vi "GEvt-Generate Unregister Log.vi"(0 "CSM Global Log Event":T4, 1 "Current State":string, 2 "Arguments":string, 6 "Name (\"\" to Use UUID)":string, 7 "Remove For Module Exit? (F)":bool, 10 "CSM:LogFilter.lvclass":refnum<class "LogFilter.lvclass">) -> (14 "CSM Global Log Event Out":T4, 16 "Event Data":T1={"Name (\"\" to Use UUID)"="", "Current State"="", "Arguments"="", "Source Message"={"‘State"="", "’Arguments"="", "’Error"={"status"=FALSE, "code"=0, "source"=""}}, "Source Module"="", "Complete(T)/Start(F)"=FALSE, "LogType"=enum."State Change", "Time Stamp"=timestamp(0 s since 1904-01-01)})   [LabVIEW 2017, in "Communicable State Machine.lvlib"]
doc: "### GEvt-Generate Unregister Log.vi\n\n-- <b>Controls</b> --\n- <b>CSM Global Log Event</b>:\n- <b>Current State</b>:\n- <b>Arguments</b>:\n- <b>Name(\"\" to use uuid)</b>:\n- <b>CSM:LogFilter.lvclass</b>:\n\n-- <b>Indicators</b> --\n- <b>CSM Global Log Event out</b>:\n- <b>event data</b>:"
uses:
  Communicable State Machine.lvlib
  GEvt-Refs.ctl
  Typedef/_CSM_GlobalLog_MSG.ctl
  Typedef/_CSM_Response Source Message.ctl
  Typedef/_CSM_GlobalLog_MSG_TYPE.ctl
  LogFilter/LogFilter.lvclass
  LogFilter/LogFilter - Check.vi
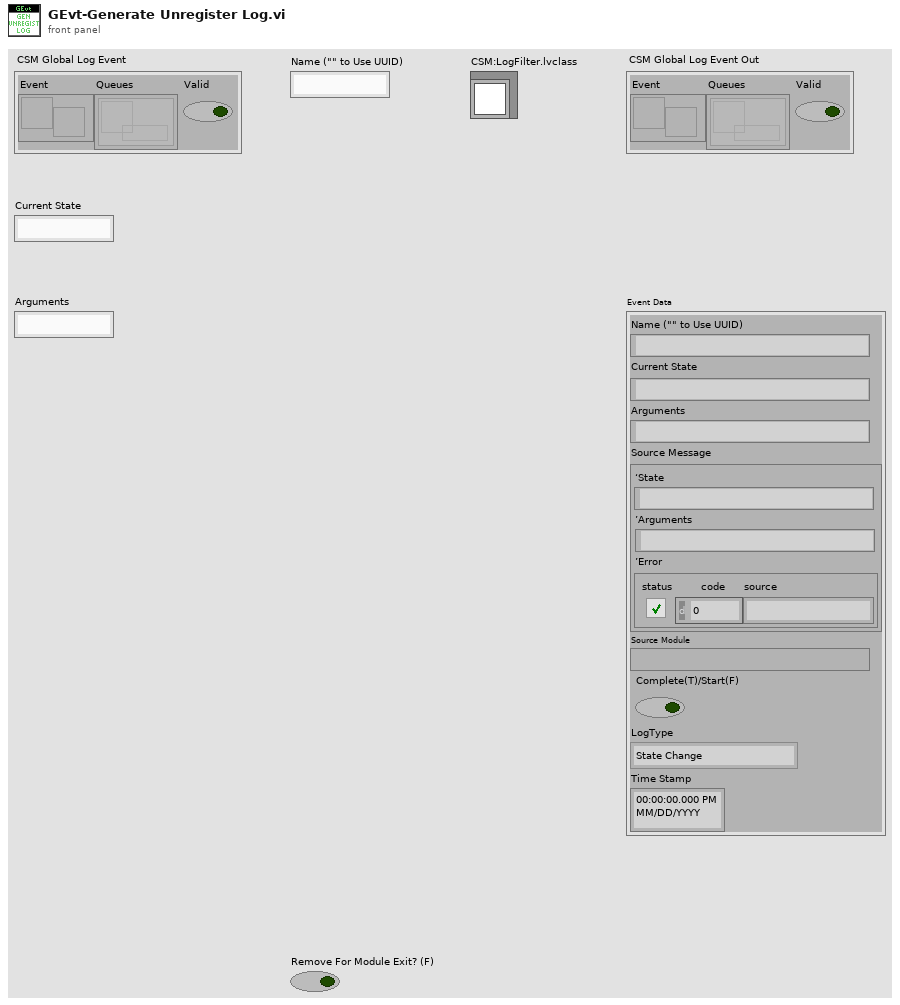
[diagram p1: front panel]
types:
  T1 = typedef "Communicable State Machine.lvlib/_CSM_GlobalLog_MSG.ctl" = cluster{"Name (\"\" to Use UUID)":string, "Current State":string, "Arguments":string, "Source Message":T2, "Source Module":string, "Complete(T)/Start(F)":bool, "LogType":T3, "Time Stamp":timestamp}
  T2 = typedef "Communicable State Machine.lvlib/_CSM_Response Source Message.ctl" = cluster{"‘State":string, "’Arguments":string, "’Error":errorcluster}
  T3 = typedef "Communicable State Machine.lvlib/_CSM_GlobalLog_MSG_TYPE.ctl" = enum16{"User Log", "State Change", "Status", "Interrupt", "Register", "Unregister", "Error Log", "Module Created", "Module Destroyed", "Async Message", "No-Rep Async Message", "Sync Message", "AsyncMsg Complete", "SyncMsg Complete"}
  T4 = typedef "Communicable State Machine.lvlib/GEvt-Refs.ctl" = cluster{"Event":refnum<user-event>, "Queues":refnum<queue>[], "Valid":bool}
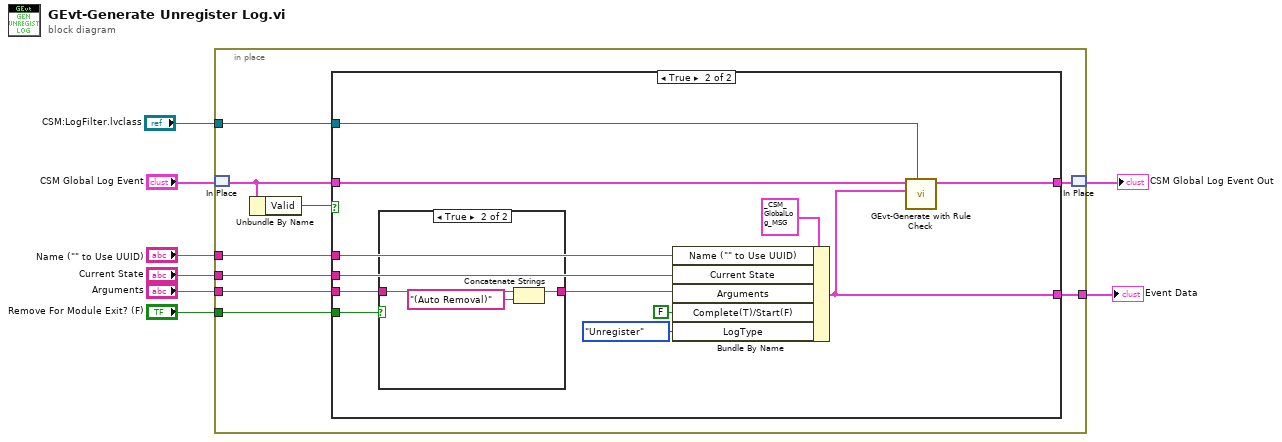
[diagram p0: block diagram]
diagram:
  n1 = in-place {
    in-place-border: [w16] -> w6
    in-place-border: "Name (\"\" to Use UUID)" -> [w15]
    in-place-border: "Current State" -> [w14]
    in-place-border: "Arguments" -> [w13]
    in-place-border: "CSM:LogFilter.lvclass" -> [w12]
    in-place-border: "Remove For Module Exit? (F)" -> [w11]
    n2 = in-place-match #1("CSM Global Log Event") -> (w10:T4)
    n3 = Unbundle By Name(w10) -> ("Valid"=w9:bool)
    n4 = case shown="True" w9 {
      tunnel: w10 -> [w18 w30]
      tunnel: [w18 w29] -> w17
      tunnel: [_ w24] -> w16
      tunnel: w15 -> [_ w26]
      tunnel: w14 -> [_ w25]
      tunnel: w13 -> [_ w19]
      tunnel: w12 -> [_ w23]
      tunnel: w11 -> [_ w21]
      frame False {
      }
      frame True {
        n5 = case shown="True" w21 {
          tunnel: [w31 w33] -> w20
          tunnel: w19 -> [w31 w34]
          frame False {
          }
          frame True {
            n6 = Concatenate Strings(w34, "(Auto Removal)" ("string")) -> (w33:string)
          }
        }
        n7 = Bundle By Name(cluster=T1 {"Name (\"\" to Use UUID)"="", "Current State"="", "Arguments"="", "Source Message"={"‘State"="", "’Arguments"="", "’Error"={"status"=FALSE, "code"=0, "source"=""}}, "Source Module"="", "Complete(T)/Start(F)"=FALSE, "LogType"=enum."State Change", "Time Stamp"=timestamp(0 s since 1904-01-01)} ("event data"), "Name (\"\" to Use UUID)"=w26, "Current State"=w25, "Arguments"=w20, "Complete(T)/Start(F)"=FALSE, "LogType"=_CSM_GlobalLog_MSG_TYPE."Unregister" ("Type")) -> (w24:T1)
        n8 = call "GEvt-Generate with Rule Check.vi"("LogFilter In"=w23, "Event Data"=w24, "CSM Global Log Event In"=w30) -> ("CSM Global Log Event Out"=w29:T4)  [unwired: 8 in]
      }
    }
    n9 = in-place-match #1(w17) -> (→"CSM Global Log Event Out":T4)
  }
  "Event Data" <- w6
